vi "Joystick_Sensitivity.vi"(1 "Deadband":dbl, 2 "Ramp":dbl, 3 "Input":dbl(slide) scale=-1.0..1.0) -> (0 "Output":dbl)   [LabVIEW 2015]
panel:
  out "Range":bool
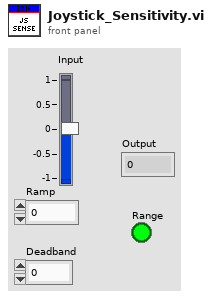
[diagram p1: front panel]
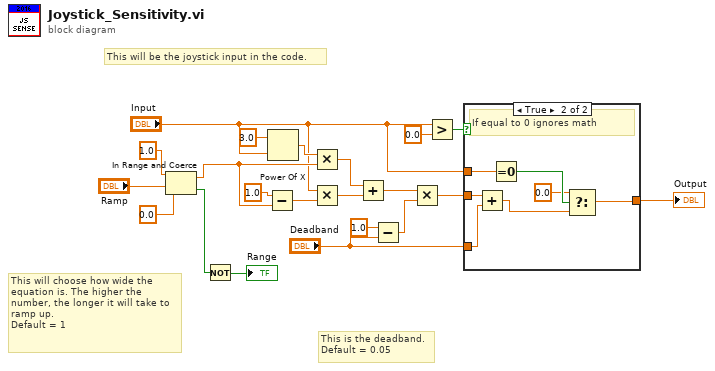
[diagram p0: block diagram]
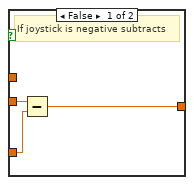
[diagram p2: hidden frame]
diagram:
  # "This will choose how wide the equation is. The higher the number, the longer it will take to ramp up.\nDefault = 1"
  # "This is the deadband.\nDefault = 0.05"
  # "This will be the joystick input in the code."
  n1 = In Range and Coerce(upper limit=1.0, x="Ramp", lower limit=0.0) -> (coerced(x)=w5:dbl, In Range?=w4:bool)
  n2 = Not(x=w4) -> (.not. x?=→"Range":bool)
  n3 = Subtract(x=1.0 ("y"), y=w5) -> (x-y=w11:dbl)
  n4 = Power Of X(1:"Input", 2:3.0 ("y")) -> (0:w12:dbl)
  n5 = Multiply(x=w12, y=w5) -> (x*y=w14:dbl)
  n6 = Multiply(x="Input", y=w11) -> (x*y=w13:dbl)
  n7 = Add(x=w14, y=w13) -> (x+y=w17:dbl)
  n8 = Subtract(x=1.0, y="Deadband") -> (x-y=w16:dbl)
  n9 = Multiply(x=w17, y=w16) -> (x*y=w20:dbl)
  n10 = Greater?(x="Input", y=0.0) -> (0:w19:bool)
  n11 = case shown="True" w19 {
    tunnel: w20 -> [w24 w31]
    tunnel: "Deadband" -> [w23 w30]
    tunnel: [w22 w27] -> w2
    tunnel: "Input" -> [_ w29]
    frame False {
      # "If joystick is negative subtracts"
      n12 = Subtract(x=w24, y=w23) -> (x-y=w22:dbl)
    }
    frame True {
      # "If equal to 0 ignores math"
      n13 = Add(x=w31, y=w30) -> (x+y=w26:dbl)
      n14 = Equal To 0?(x=w29) -> (x = 0?=w28:bool)
      n15 = Select(t=0.0, s=w28, f=w26) -> (s? t:f=w27:dbl)
    }
  }
  "Output" <- w2
